vi "lsl get channel format.vi"(8 "error in (no error)":errorcluster, 11 "streaminfo":T2) -> (0 "error out":errorcluster, 3 "channel_format":T1=1 items=["cft_float32"=1, "cft_double64"=2, "cft_string"=3, "cft_int32"=4, "cft_int16"=5, "cft_int8"=6, "cft_int64"=7, "cft_undefined"=0])   [LabVIEW 2018, in "liblsl-LabVIEW.lvlib"]
doc: "extern LIBLSL_C_API lsl_channel_format_t lsl_get_channel_format(lsl_streaminfo info);"
uses:
  <userlib>/liblsl-LabVIEW/liblsl-LabVIEW.lvlib
  <userlib>/liblsl-LabVIEW/Custom Controls/lsl_streaminfo.ctl
  <userlib>/liblsl-LabVIEW/Custom Controls/lsl_channel_format.ctl
  <userlib>/liblsl-LabVIEW/liblsl64.dll
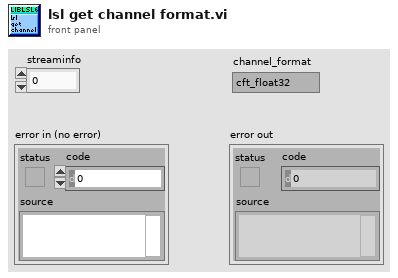
[diagram p1: front panel]
types:
  T1 = typedef "liblsl-LabVIEW.lvlib/lsl_channel_format.ctl" = u32
  T2 = typedef "liblsl-LabVIEW.lvlib/lsl_streaminfo.ctl" = u64
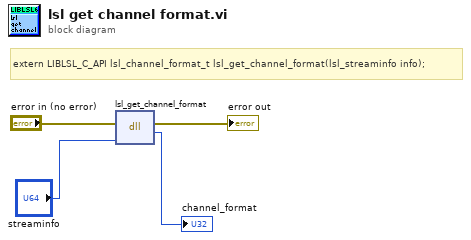
[diagram p0: block diagram]
diagram:
  # "extern LIBLSL_C_API lsl_channel_format_t lsl_get_channel_format(lsl_streaminfo info);"
  n1 = dll-call lib="C:/Program Files/National Instruments/LabVIEW 2018/user.lib/liblsl-LabVIEW/liblsl64.dll" fn="lsl_get_channel_format"(error in="error in (no error)", "info"="streaminfo") -> (error out=→"error out":errorcluster, "return type"=→"channel_format":u32)  [unwired: 3 in, 1 out]
